vi "e.gate HighSpeedPort Decode Data Type.vi"(8 "error in (no errro)":errorcluster, 9 "Precision":i16, 10 "DataTypeIndex":T1, 11 "data in (binary)":u8[](array[numeric])) -> (0 "error out":errorcluster, 1 "ByteCount":i32, 2 "DataType":string, 3 "value (double)":dbl format="%#_8f")   [LabVIEW 2016]
doc: "This VI is used to decode a binary data arry to a double value using channel data from the configuration cluster."
uses:
  e.gate Data Type.ctl
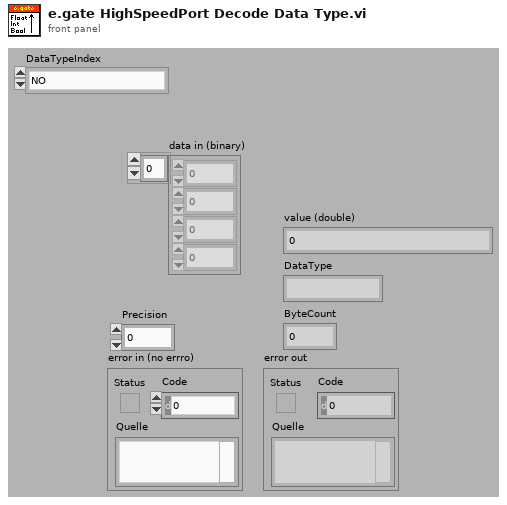
[diagram p1: front panel]
types:
  T1 = typedef "e.gate Data Type.ctl" = enum16{"NO", "BOOL", "SINT8", "USINT8", "SINT16", "USINT16", "SINT32", "USINT32", "FLOAT", "SET8", "SET16", "SET32", "DOUBLE", "SINT64", "USINT64", "SET64"}
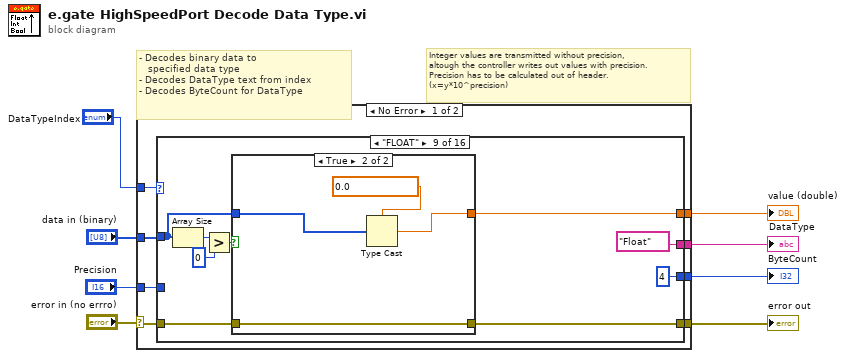
[diagram p0: block diagram]
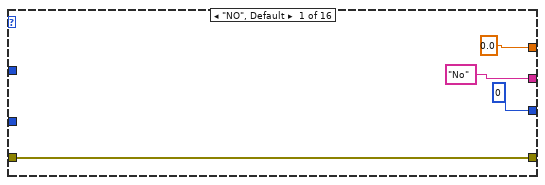
[diagram p2: hidden frame]
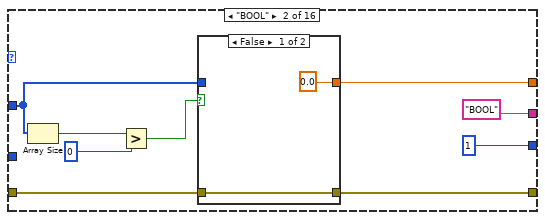
[diagram p3: hidden frame]
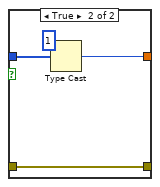
[diagram p4: hidden frame]
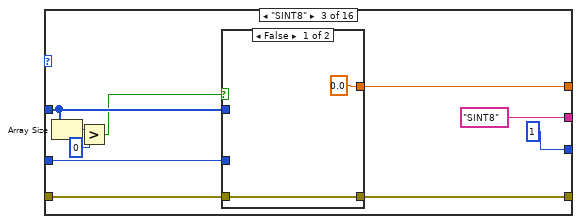
[diagram p5: hidden frame]
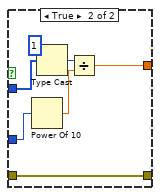
[diagram p6: hidden frame]
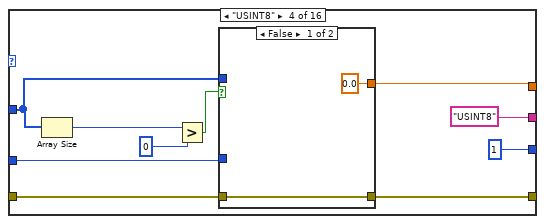
[diagram p7: hidden frame]
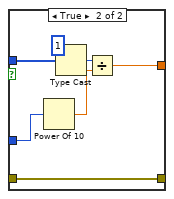
[diagram p8: hidden frame]
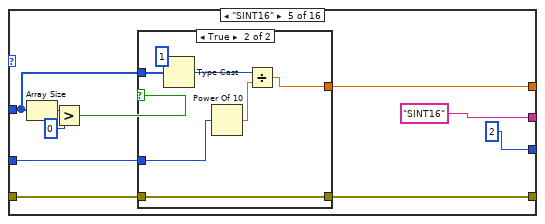
[diagram p9: hidden frame]
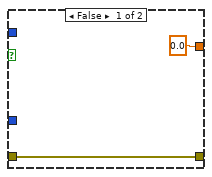
[diagram p10: hidden frame]
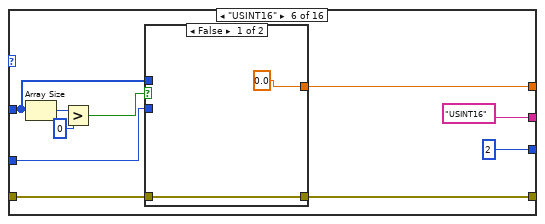
[diagram p11: hidden frame]
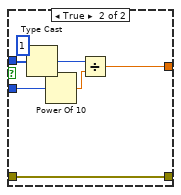
[diagram p12: hidden frame]
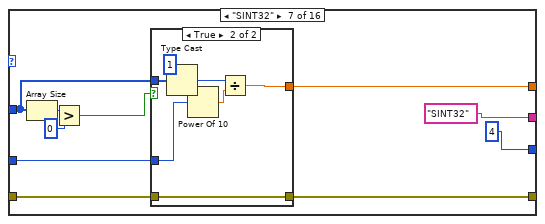
[diagram p13: hidden frame]
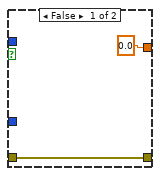
[diagram p14: hidden frame]
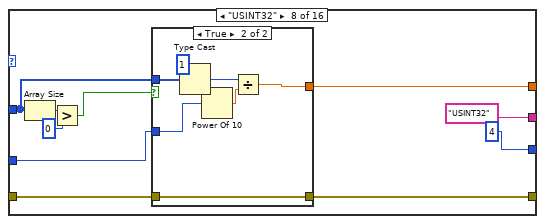
[diagram p15: hidden frame]
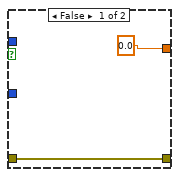
[diagram p16: hidden frame]
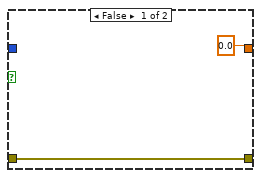
[diagram p17: hidden frame]
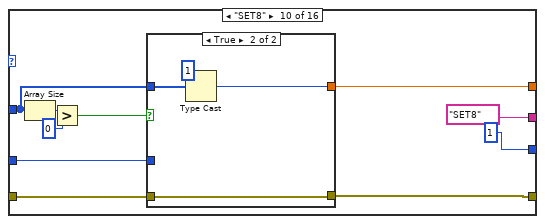
[diagram p18: hidden frame]
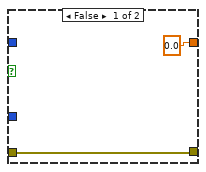
[diagram p19: hidden frame]
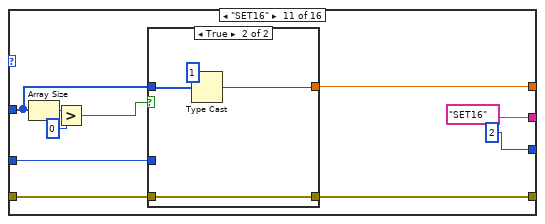
[diagram p20: hidden frame]
diagram:
  # "Integer values are transmitted without precision,\naltough the controller writes out values with precision.\nPrecision has to be calculated out of header.\n(x=y*10^precision)"
  # "- Decodes binary data to\n   specified data type\n- Decodes DataType text from index\n- Decodes ByteCount for DataType"
  n1 = case shown="No Error" "error in (no errro)" {
    selector: "error in (no errro)" -> [w10 w282]
    tunnel: "DataTypeIndex" -> [w16 _]
    tunnel: [w15 0.0] -> w8
    tunnel: "data in (binary)" -> [w14 _]
    tunnel: "Precision" -> [w13 _]
    tunnel: [w12 ""] -> w5
    tunnel: [w11 0 ("Precision")] -> w4
    tunnel: [w9 w282] -> w3
    frame No Error {
      n2 = case shown="\"FLOAT\"" w16 {
        tunnel: ["No" "BOOL" "SINT8" "USINT8" "SINT16" "USINT16" "SINT32" "USINT32" "Float" "SET8" "SET16" "SET32" "SET64" "DOUBLE" "USINT64" "SINT64"] -> w12
        tunnel: w14 -> [_ w24 w41 w57 w77 w99 w118 w136 w154 w167 w186 w204 w220 w232 w244 w263]
        tunnel: [i16 0 ("Precision") i16 1 ("Precision") 1 1 ("Precision") 2 ("Precision") 2 ("Precision") 4 ("Precision") 4 ("Precision") 4 ("Precision") 1 ("Precision") 2 ("Precision") 4 ("Precision") 8 ("Precision") i16 8 ("Precision") 8 ("Precision") 8 ("Precision")] -> w11
        tunnel: w13 -> [_ _ w44 w59 w79 w98 w117 w135 _ w170 w185 w203 w219 _ w245 w264]
        tunnel: [0.0 w23 w42 w58 w78 w97 w115 w134 w153 w169 w184 w201 w217 w231 w246 w265] -> w15
        tunnel: w10 -> [w17 w22 w37 w56 w75 w93 w113 w132 w151 w165 w182 w198 w214 w230 w247 w266]
        tunnel: [w17 w21 w36 w55 w74 w94 w112 w131 w150 w166 w181 w197 w213 w229 w248 w267] -> w9
        frame "NO", Default {
        }
        frame "BOOL" {
          n3 = Array Size(array=w24) -> (size(s)=w27:i32)
          n4 = Greater?(x=w27, y=0) -> (0:w25:bool)
          n5 = case shown="False" w25 {
            tunnel: w24 -> [_ w34]
            tunnel: [0.0 w33] -> w23
            tunnel: w22 -> [w30 w32]
            tunnel: [w30 w32] -> w21
            frame False {
            }
            frame True {
              n6 = Type Cast(type=u8 1, x=w34) -> (*(type *) &x=w33:u8)
            }
          }
        }
        frame "SINT8" {
          n7 = Array Size(array=w41) -> (size(s)=w40:i32)
          n8 = Greater?(x=w40, y=0) -> (0:w38:bool)
          n9 = case shown="False" w38 {
            tunnel: w44 -> [_ w50]
            tunnel: [0.0 w49] -> w42
            tunnel: w41 -> [_ w52]
            tunnel: w37 -> [w46 w48]
            tunnel: [w46 w48] -> w36
            frame False {
            }
            frame True {
              n10 = Power Of 10(x=w50) -> (10^x=w51:dbl)
              n11 = Type Cast(type=i8 1, x=w52) -> (*(type *) &x=w53:i8)
              n12 = Divide(x=w53, y=w51) -> (x/y=w49:dbl)
            }
          }
        }
        frame "USINT8" {
          n13 = Array Size(array=w57) -> (size(s)=w60:i32)
          n14 = Greater?(x=w60, y=0) -> (0:w62:bool)
          n15 = case shown="False" w62 {
            tunnel: w59 -> [_ w70]
            tunnel: [0.0 w68] -> w58
            tunnel: w57 -> [_ w71]
            tunnel: w56 -> [w65 w67]
            tunnel: [w65 w67] -> w55
            frame False {
            }
            frame True {
              n16 = Power Of 10(x=w70) -> (10^x=w69:dbl)
              n17 = Type Cast(type=u8 1, x=w71) -> (*(type *) &x=w72:u8)
              n18 = Divide(x=w72, y=w69) -> (x/y=w68:dbl)
            }
          }
        }
        frame "SINT16" {
          n19 = Array Size(array=w77) -> (size(s)=w82:i32)
          n20 = Greater?(x=w82, y=0) -> (0:w80:bool)
          n21 = case shown="True" w80 {
            tunnel: [0.0 w87] -> w78
            tunnel: w79 -> [_ w89]
            tunnel: w77 -> [_ w88]
            tunnel: w75 -> [w84 w86]
            tunnel: [w84 w86] -> w74
            frame False {
            }
            frame True {
              n22 = Type Cast(type=i16 1, x=w88) -> (*(type *) &x=w91:i16)
              n23 = Power Of 10(x=w89) -> (10^x=w90:dbl)
              n24 = Divide(x=w91, y=w90) -> (x/y=w87:dbl)
            }
          }
        }
        frame "USINT16" {
          n25 = Array Size(array=w99) -> (size(s)=w101:i32)
          n26 = Greater?(x=w101, y=0) -> (0:w95:bool)
          n27 = case shown="False" w95 {
            tunnel: [0.0 w106] -> w97
            tunnel: w99 -> [_ w108]
            tunnel: w98 -> [_ w107]
            tunnel: [w103 w105] -> w94
            tunnel: w93 -> [w103 w105]
            frame False {
            }
            frame True {
              n28 = Type Cast(type=u16 1, x=w108) -> (*(type *) &x=w111:u16)
              n29 = Power Of 10(x=w107) -> (10^x=w110:dbl)
              n30 = Divide(x=w111, y=w110) -> (x/y=w106:dbl)
            }
          }
        }
        frame "SINT32" {
          n31 = Array Size(array=w118) -> (size(s)=w120:i32)
          n32 = Greater?(x=w120, y=0) -> (0:w116:bool)
          n33 = case shown="True" w116 {
            tunnel: [0.0 w125] -> w115
            tunnel: w118 -> [_ w127]
            tunnel: w117 -> [_ w126]
            tunnel: w113 -> [w122 w124]
            tunnel: [w122 w124] -> w112
            frame False {
            }
            frame True {
              n34 = Type Cast(type=1, x=w127) -> (*(type *) &x=w130:i32)
              n35 = Power Of 10(x=w126) -> (10^x=w129:dbl)
              n36 = Divide(x=w130, y=w129) -> (x/y=w125:dbl)
            }
          }
        }
        frame "USINT32" {
          n37 = Array Size(array=w136) -> (size(s)=w139:i32)
          n38 = Greater?(x=w139, y=0) -> (0:w137:bool)
          n39 = case shown="True" w137 {
            tunnel: [0.0 w144] -> w134
            tunnel: w136 -> [_ w146]
            tunnel: w135 -> [_ w145]
            tunnel: w132 -> [w141 w143]
            tunnel: [w141 w143] -> w131
            frame False {
            }
            frame True {
              n40 = Type Cast(type=u32 1, x=w146) -> (*(type *) &x=w149:u32)
              n41 = Power Of 10(x=w145) -> (10^x=w148:dbl)
              n42 = Divide(x=w149, y=w148) -> (x/y=w144:dbl)
            }
          }
        }
        frame "FLOAT" {
          n43 = Array Size(array=w154) -> (size(s)=w157:i32)
          n44 = Greater?(x=w157, y=0) -> (0:w155:bool)
          n45 = case shown="True" w155 {
            tunnel: [0.0 w164] -> w153
            tunnel: w154 -> [_ w163]
            tunnel: w151 -> [w159 w162]
            tunnel: [w159 w162] -> w150
            frame False {
            }
            frame True {
              n46 = Type Cast(type=sgl 0.0, x=w163) -> (*(type *) &x=w164:sgl)
            }
          }
        }
        frame "SET8" {
          n47 = Array Size(array=w167) -> (size(s)=w173:i32)
          n48 = Greater?(x=w173, y=0) -> (0:w171:bool)
          n49 = case shown="True" w171 {
            tunnel: [0.0 w179] -> w169
            tunnel: w170 -> [_ _]
            tunnel: w167 -> [_ w178]
            tunnel: [w175 w177] -> w166
            tunnel: w165 -> [w175 w177]
            frame False {
            }
            frame True {
              n50 = Type Cast(type=i8 1, x=w178) -> (*(type *) &x=w179:i8)
            }
          }
        }
        frame "SET16" {
          n51 = Array Size(array=w186) -> (size(s)=w189:i32)
          n52 = Greater?(x=w189, y=0) -> (0:w187:bool)
          n53 = case shown="True" w187 {
            tunnel: [0.0 w194] -> w184
            tunnel: w186 -> [_ w195]
            tunnel: w185 -> [_ _]
            tunnel: w182 -> [w191 w193]
            tunnel: [w191 w193] -> w181
            frame False {
            }
            frame True {
              n54 = Type Cast(type=i16 1, x=w195) -> (*(type *) &x=w194:i16)
            }
          }
        }
        frame "SET32" {
          n55 = Array Size(array=w204) -> (size(s)=w206:i32)
          n56 = Greater?(x=w206, y=0) -> (0:w202:bool)
          n57 = case shown="True" w202 {
            tunnel: [0.0 w210] -> w201
            tunnel: w204 -> [_ w211]
            tunnel: w203 -> [_ _]
            tunnel: w198 -> [w207 w209]
            tunnel: [w207 w209] -> w197
            frame False {
            }
            frame True {
              n58 = Type Cast(type=1, x=w211) -> (*(type *) &x=w210:i32)
            }
          }
        }
        frame "SET64" {
          n59 = Array Size(array=w220) -> (size(s)=w222:i32)
          n60 = Greater?(x=w222, y=0) -> (0:w218:bool)
          n61 = case shown="True" w218 {
            tunnel: [0.0 w226] -> w217
            tunnel: w220 -> [_ w227]
            tunnel: w219 -> [_ _]
            tunnel: w214 -> [w223 w225]
            tunnel: [w223 w225] -> w213
            frame False {
            }
            frame True {
              n62 = Type Cast(type=u64 1, x=w227) -> (*(type *) &x=w226:u64)
            }
          }
        }
        frame "DOUBLE" {
          n63 = Array Size(array=w232) -> (size(s)=w235:i32)
          n64 = Greater?(x=w235, y=0) -> (0:w233:bool)
          n65 = case shown="True" w233 {
            tunnel: [0.0 w241] -> w231
            tunnel: w232 -> [_ w242]
            tunnel: w230 -> [w238 w240]
            tunnel: [w238 w240] -> w229
            frame False {
            }
            frame True {
              n66 = Type Cast(type=1.0, x=w242) -> (*(type *) &x=w241:dbl)
            }
          }
        }
        frame "USINT64" {
          n67 = Array Size(array=w244) -> (size(s)=w251:i32)
          n68 = Greater?(x=w251, y=0) -> (0:w253:bool)
          n69 = case shown="True" w253 {
            tunnel: [0.0 w257] -> w246
            tunnel: w244 -> [_ w259]
            tunnel: w245 -> [_ w258]
            tunnel: w247 -> [w254 w256]
            tunnel: [w254 w256] -> w248
            frame False {
            }
            frame True {
              n70 = Type Cast(type=u64 1, x=w259) -> (*(type *) &x=w262:u64)
              n71 = Power Of 10(x=w258) -> (10^x=w261:dbl)
              n72 = Divide(x=w262, y=w261) -> (x/y=w257:dbl)
            }
          }
        }
        frame "SINT64" {
          n73 = Array Size(array=w263) -> (size(s)=w270:i32)
          n74 = Greater?(x=w270, y=0) -> (0:w272:bool)
          n75 = case shown="True" w272 {
            tunnel: [0.0 w276] -> w265
            tunnel: w263 -> [_ w278]
            tunnel: w264 -> [_ w277]
            tunnel: w266 -> [w273 w275]
            tunnel: [w273 w275] -> w267
            frame False {
            }
            frame True {
              n76 = Type Cast(type=i64 1, x=w278) -> (*(type *) &x=w281:i64)
              n77 = Power Of 10(x=w277) -> (10^x=w280:dbl)
              n78 = Divide(x=w281, y=w280) -> (x/y=w276:dbl)
            }
          }
        }
      }
    }
    frame Error {
    }
  }
  "value (double)" <- w8
  "DataType" <- w5
  "ByteCount" <- w4
  "error out" <- w3
